vi "ErrorHandler.vi"(5 "Clear Error":bool, 6 "Error In":errorcluster, 9 "Name":string) -> (0 "Error Out":errorcluster, 3 "Named Error Out":T1)   [LabVIEW 2014]
uses:
  Controls/NamedError.ctl
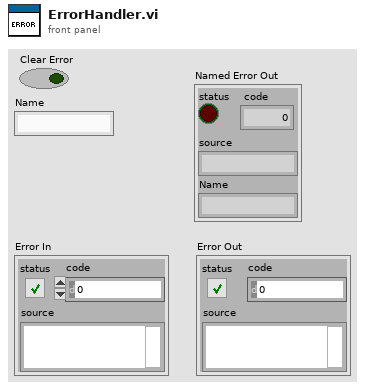
[diagram p1: front panel]
types:
  T1 = typedef "NamedError.ctl" = cluster{"status":bool, "code":i32, "source":string, "Name":string}
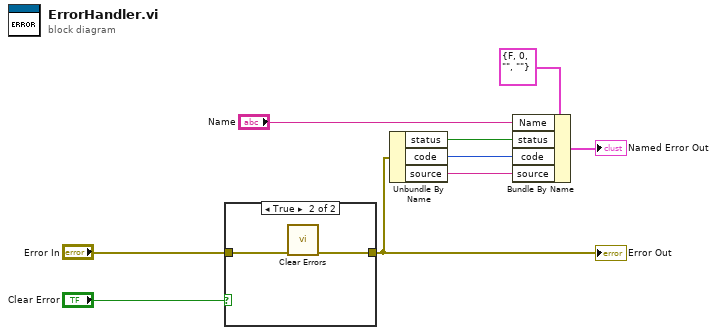
[diagram p0: block diagram]
diagram:
  n1 = case shown="True" "Clear Error" {
    tunnel: "Error In" -> [w10 w12]
    tunnel: [w10 w11] -> w1
    frame False {
    }
    frame True {
      n2 = call <vilib>:"Clear Errors.vi"("error in (no error)"=w12) -> ("error out"=w11:errorcluster)  [unwired: 5 in, 1 out]
    }
  }
  "Error Out" <- w1
  n3 = Unbundle By Name(w1) -> ("status"=w7:bool, "code"=w6:i32, "source"=w5:string)
  n4 = Bundle By Name(cluster=T1 {"status"=FALSE, "code"=0, "source"="", "Name"=""} ("Named Error Out"), "Name"="Name", "status"=w7, "code"=w6, "source"=w5) -> (→"Named Error Out":T1)
